vi "Read DeviceID.vi"(8 "error in (no error)":errorcluster, 11 "2936r in":refnum<class "2936r.lvclass">) -> (0 "error out":errorcluster, 2 "DeviceID":string, 3 "2936r out":refnum<class "2936r.lvclass">)   [LabVIEW 2018, in "2936r.lvlib" / "2936r.lvclass"]
uses:
  2936r.lvclass
  2936r.lvclass/2936r.ctl
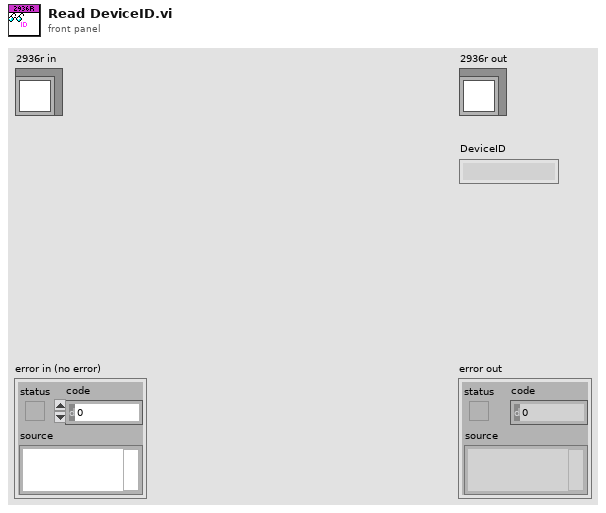
[diagram p1: front panel]
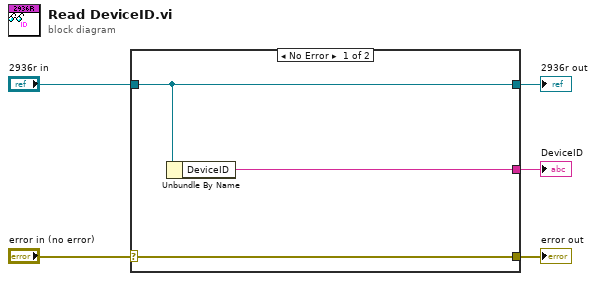
[diagram p0: block diagram]
diagram:
  n1 = case shown="No Error" "error in (no error)" {
    selector: "error in (no error)" -> [w8 w9]
    tunnel: [w8 w9] -> w4
    tunnel: [w7 w10] -> w2
    tunnel: "2936r in" -> [w7 w10]
    tunnel: [w6 _] -> w1
    frame No Error {
      n2 = Unbundle By Name(w7) -> ("DeviceID"=w6:string)
    }
    frame Error {
    }
  }
  "error out" <- w4
  "2936r out" <- w2
  "DeviceID" <- w1
